vi "Test_GPS_Listen.vi"() -> ()   [LabVIEW 2016]
uses:
  Libraries/OBJ-Serial/Controls/Cmd_Rx.ctl
  Libraries/OBJ-GPS/Controls/typedef_cluster_GPGGA.ctl
  Libraries/OBJ-GPS/Controls/typedef_enum_DirLat.ctl
  Libraries/OBJ-GPS/Controls/typedef_enum_DirLong.ctl
  Libraries/OBJ-GPS/Controls/typedef_enum_GPS_Quality.ctl
  Libraries/OBJ-GPS/Controls/typedef_cluster_GPRMC.ctl
  Libraries/OBJ-GPS/Controls/typedef_cluster_GPVTG.ctl
  Libraries/OBJ-GPS/Controls/typedef_enum_Mode.ctl
  Libraries/OBJ-Serial/Controls/PortConfig.ctl
  Libraries/OBJ-Serial/Serial_G.lvlib
  Libraries/OBJ-GPS/NMEA.lvlib
panel:
  out "GPGSV":string
  out "GPGSA":string
  out "Resp":string
  in  "ms_delay":u32=1
  out "GPVTG":string
  out "GPRMC":string
  out "GPGGA":string
  out "$GPVTG":T1={"True Course over Ground"=0.0, "Magnetic Course over Ground"=0.0, "Speed over Ground in knots"=0.0, "Speed over Ground in km/h"=1.0, "Mode"=""} {"Speed over Ground in km/h" format="%.02f [km/h]"; "Speed over Ground in knots" format="%.02f [kts]"; "Magnetic Course over Ground" format="%.02f [deg]"; "True Course over Ground" format="%.02f [deg]"}
  out "$GPRMC":T3={"TimeStamp"=timestamp(0 s since 1904-01-01), "Validity"=FALSE, "Latitude"=0.0, "Latitude-Direction"=enum."North", "Longitude"=0.0, "Longitude-Direction"=enum."East", "Speed in knots"=0.0, "True course"=0.0, "Date Stamp"=timestamp(0 s since 1904-01-01), "Magnetic Variation (East/West)"=0.0} {"Magnetic Variation (East/West)" format="%.02f [deg]"; "Date Stamp" format="%<%x>T"; "True course" format="%.02f [deg]"; "Speed in knots" format="%.02f [kts]"; "Longitude" format="%0.4f [long]"; "Latitude" format="%.04f [lat]"; "TimeStamp" format="%<%.2X>T"}
  out "$GPGGA":T6={"TimeStamp"=timestamp(0 s since 1904-01-01), "Latitude"=0.0, "Latitude-Direction"=enum."", "Longitude"=1.0, "Longitude-Direction"=enum."", "GPS-Quality"=enum."GPS fix", "Number of Satellites"=0, "Horizontal Dilution of Precision"=0.0, "Altitude above Mean-Sea-Level"=0.0, "Geoidal separation"=0.0, "Time since last DGPS update"=0.0, "DGPS reference station ID"=0} {"Time since last DGPS update" format="%.02f [s]"; "Geoidal separation" format="%.02f [m]"; "Altitude above Mean-Sea-Level" format="%.02f [m]"; "Horizontal Dilution of Precision" format="%.02f [HDOP]"; "Longitude" format="%0.4f [long]"; "Latitude" format="%.04f [lat]"; "TimeStamp" format="%<%.2X>T"}
  out "CheckSumOk?":bool
  in  "Timeout":u32=1000
  in  "Exit":bool
  out "Port?":bool
  out "Read":T8
  in  "error in":errorcluster
  in  "Port":string="COM13"
  out "error out":errorcluster
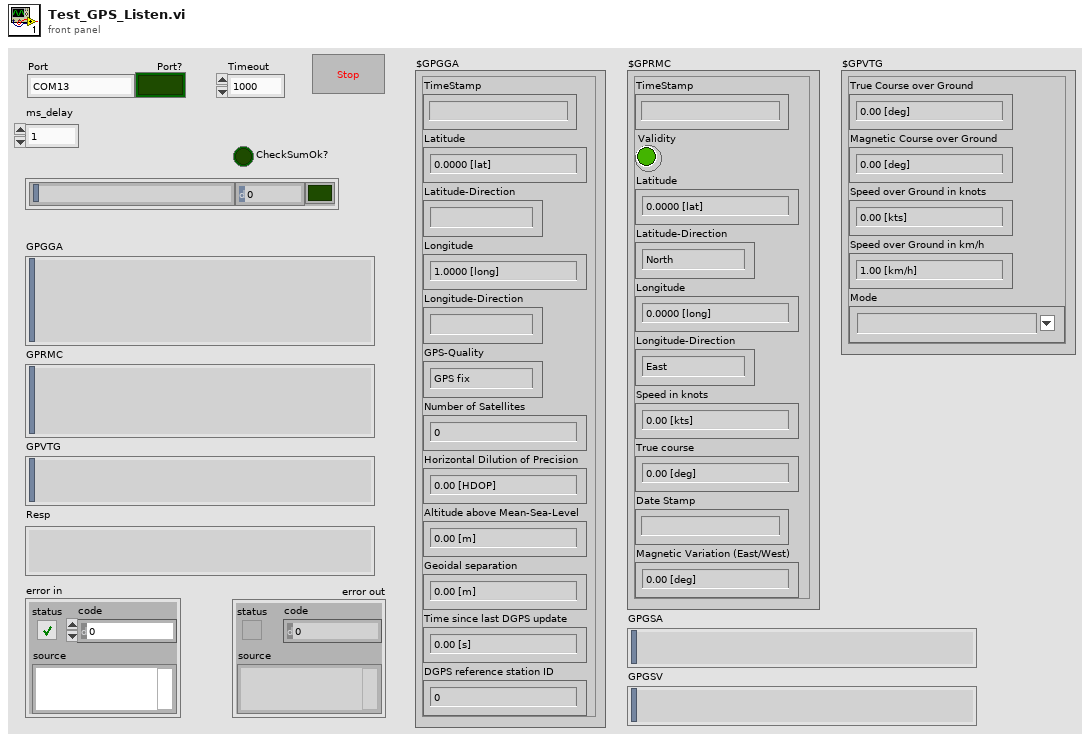
[diagram p1: front panel]
types:
  T1 = typedef "NMEA.lvlib/typedef_cluster_GPVTG.ctl" = cluster{"True Course over Ground":dbl, "Magnetic Course over Ground":dbl, "Speed over Ground in knots":dbl, "Speed over Ground in km/h":dbl, "Mode":T2}
  T2 = typedef "NMEA.lvlib/typedef_enum_Mode.ctl" = string
  T3 = typedef "NMEA.lvlib/typedef_cluster_GPRMC.ctl" = cluster{"TimeStamp":timestamp, "Validity":bool, "Latitude":dbl, "Latitude-Direction":T4, "Longitude":dbl, "Longitude-Direction":T5, "Speed in knots":dbl, "True course":dbl, "Date Stamp":timestamp, "Magnetic Variation (East/West)":dbl}
  T4 = typedef "NMEA.lvlib/typedef_enum_DirLat.ctl" = enum16{"", "North", "South"}
  T5 = typedef "NMEA.lvlib/typedef_enum_DirLong.ctl" = enum16{"", "East", "West"}
  T6 = typedef "NMEA.lvlib/typedef_cluster_GPGGA.ctl" = cluster{"TimeStamp":timestamp, "Latitude":dbl, "Latitude-Direction":T4, "Longitude":dbl, "Longitude-Direction":T5, "GPS-Quality":T7, "Number of Satellites":i32, "Horizontal Dilution of Precision":dbl, "Altitude above Mean-Sea-Level":dbl, "Geoidal separation":dbl, "Time since last DGPS update":dbl, "DGPS reference station ID":i32}
  T7 = typedef "NMEA.lvlib/typedef_enum_GPS_Quality.ctl" = enum16{"Invalid", "GPS fix", "DGPS fix"}
  T8 = typedef "Serial_G.lvlib/Cmd_Rx.ctl" = cluster{"Read":string, "ExecTime (ms)":i32, "Timeout?":bool}
  T9 = typedef "Serial_G.lvlib/PortConfig.ctl" = cluster{"Baud rate":u32, "Parity":enum16{"None", "Odd", "Even", "Mark", "Space"}, "Data bits":u16, "Stop bits":u16, "Flow control":u16}
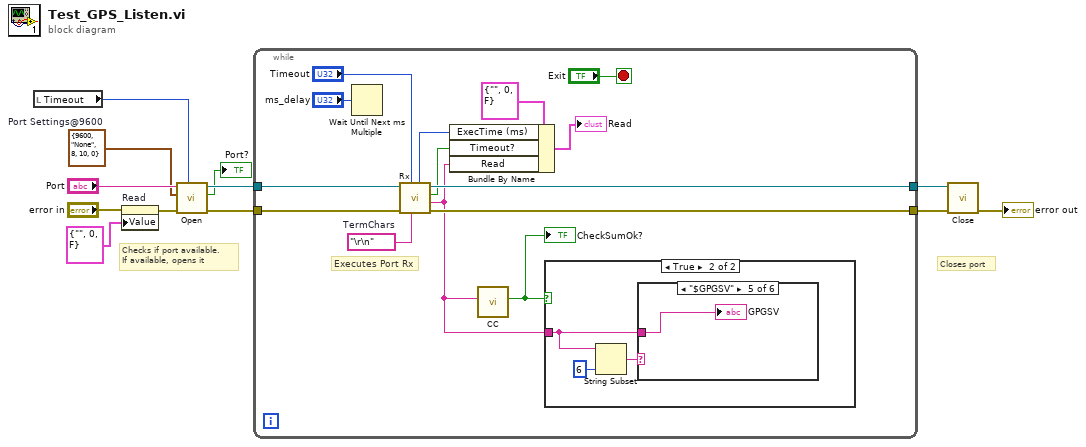
[diagram p0: block diagram]
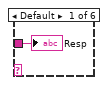
[diagram p3: hidden frame]
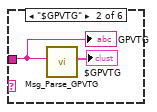
[diagram p4: hidden frame]
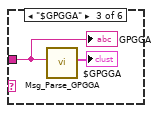
[diagram p5: hidden frame]
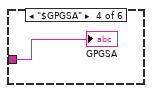
[diagram p6: hidden frame]
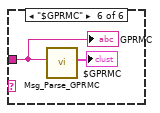
[diagram p7: hidden frame]
diagram:
  w2 = T9 {"Baud rate"=9600, "Parity"=enum."None", "Data bits"=8, "Stop bits"=10, "Flow control"=0}  # Port Settings@9600
  # "Closes port"
  # "Checks if port available.\nIf available, opens it"
  n1 = local read "Timeout"() -> (w1:u32)
  n2 = property on="Read" class="Clust (strict)"(error in="error in", "Value"=T8 {"Read"="", "ExecTime (ms)"=0, "Timeout?"=FALSE} ("Read")) -> (error out=w5:errorcluster)  [unwired: 1 in, 1 out]
  n3 = call "Open.vi"("Timeout (3000)"=w1, "error in"=w5, "ConfigPort (9600,0,8,1)"=w2, "Port(Alias)"="Port") -> ("error out"=w12:errorcluster, "PortFound?"=→"Port?":bool, "VISA out"=w11:refnum<visa-resource-name>)  [unwired: 4 in, 1 out]
  n4 = while {
    tunnel: w11 -> [w25]
    tunnel: [w24] -> w10
    tunnel: w12 -> [w26]
    tunnel: [w23] -> w8
    stop <- "Exit" stop-if-true
    w19 = "\r\n"  # TermChars
    # "Executes Port Rx"
    n5 = Wait Until Next ms Multiple(millisecond multiple="ms_delay") -> ()  [unwired: 1 out]
    n6 = call "Rx.vi"("Wait for? (\\r\\n)"=w19, "Timeout_ms (3000)"="Timeout", "error in"=w26, "VISA in"=w25) -> ("error out"=w23:errorcluster, "Response"=w16:string, "Timeout?"=w21:bool, "VISA out"=w24:refnum<visa-resource-name>, "ExecTime(ms)"=w20:i32)  [unwired: 3 in]
    n7 = Bundle By Name(cluster=T8 {"Read"="", "ExecTime (ms)"=0, "Timeout?"=FALSE} ("Read"), "ExecTime (ms)"=w20, "Timeout?"=w21, "Read"=w16) -> (→"Read":T8)
    n8 = call "CC.vi"("Sentence"=w16) -> ("CheckSumOk?"=w15:bool)  [unwired: 9 in, 1 out]
    "CheckSumOk?" <- w15
    n9 = case shown="True" w15 {
      tunnel: w16 -> [_ w27]
      frame False {
      }
      frame True {
        n10 = String Subset(string=w27, length (rest)=6 ("length (rest)")) -> (substring=w28:string)  [unwired: 1 in]
        n11 = case shown="\"$GPGSV\"" w28 {
          tunnel: w27 -> [w30 w31 w33 w35 w36 w37]
          frame Default {
            "Resp" <- w30
          }
          frame "$GPVTG" {
            n12 = call "Msg_Parse_GPVTG.vi"("$GPVTG-message_IN"=w31) -> ("$GPVTG-message_OUT"=→"$GPVTG":T1)  [unwired: 9 in, 1 out]
            "GPVTG" <- w31
          }
          frame "$GPGGA" {
            n13 = call "Msg_Parse_GPGGA.vi"("$GPGGA-message_IN"=w33) -> ("$GPGGA-message_OUT"=→"$GPGGA":T6)  [unwired: 9 in, 1 out]
            "GPGGA" <- w33
          }
          frame "$GPGSA" {
            "GPGSA" <- w35
          }
          frame "$GPGSV" {
            "GPGSV" <- w36
          }
          frame "$GPRMC" {
            n14 = call "Msg_Parse_GPRMC.vi"("$GPRMC-message_IN"=w37) -> ("$GPRMC-message_OUT"=→"$GPRMC":T3)  [unwired: 9 in, 1 out]
            "GPRMC" <- w37
          }
        }
      }
    }
  }
  n15 = call "Close.vi"("error in"=w8, "VISA in"=w10) -> ("error out"=→"error out":errorcluster)  [unwired: 9 in]
